vi "Logic.vi"(8 "error in (no error)":errorcluster, 11 "CIFPlugin in":refnum<class "Template_Plugin.lvclass">) -> (0 "error out":errorcluster, 3 "CIFPlugin out":refnum<class "Template_Plugin.lvclass">)   [LabVIEW 2021, in "Template_Plugin.lvclass"]
uses:
  Template_Plugin.lvclass
  <vilib>/CIF Foundation/CIF Core/CIFCore/Class/CIFCorePlugin.lvclass
  Common/Typedef/Channels.ctl
  Common/Template_Common.lvlib
  C:/Program Files/National Instruments/LabVIEW 2021/vi.lib/CIF Foundation/CIF Core/CIFCore/Class/CIFCorePlugin.lvclass
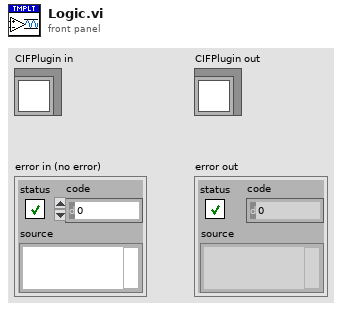
[diagram p1: front panel]
types:
  T1 = typedef "Template_Common.lvlib/Channels.ctl" = enum16{"doubleout", "doublein1", "doublein2", "uint_out", "uint_in"}
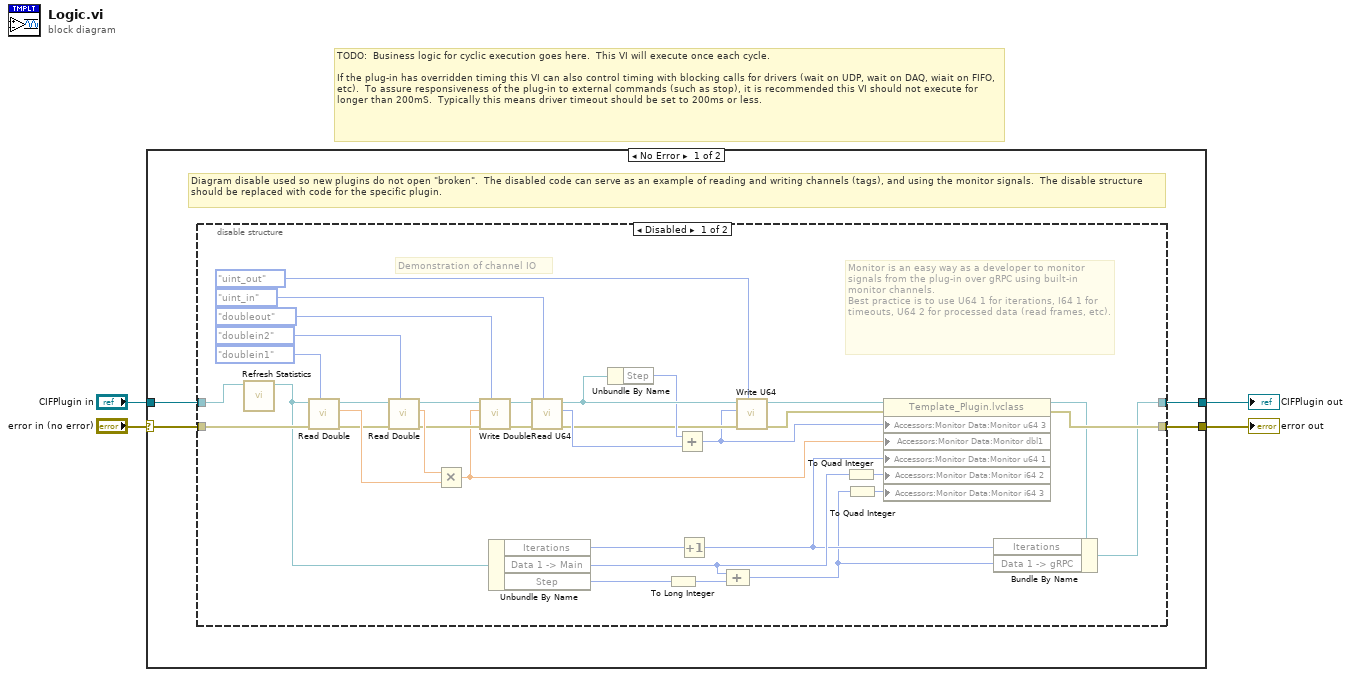
[diagram p0: block diagram]
diagram:
  # "TODO:  Business logic for cyclic execution goes here.  This VI will execute once each cycle.  \n\nIf the plug-in has overridden timing this VI can also control timing with blocking calls for drivers (wait on UDP, wait on DAQ, wiait on FIFO, etc).  To assure responsiveness of the plug-in to external commands (such as stop), it is recommended this VI should not execute for longer than 200mS.  Typically this means driver timeout should be set to 200ms or less."
  n1 = case shown="No Error" "error in (no error)" {
    selector: "error in (no error)" -> [w5 w47]
    tunnel: [w8 w47] -> w2
    tunnel: [w7 w46] -> w1
    tunnel: "CIFPlugin in" -> [w6 w46]
    frame No Error {
      # "Diagram disable used so new plugins do not open \"broken\".  The disabled code can serve as an example of reading and writing channels (tags), and using the monitor signals.  The disable structure should be replaced with code for the specific plugin."
      n2 = disable-structure shown="Disabled" {
        disable-tunnel: [w43 w44] -> w8
        disable-tunnel: [w36 w45] -> w7
        disable-tunnel: w6 -> [w10 w45]
        disable-tunnel: w5 -> [w16 w44]
        frame Disabled {
          # "Demonstration of channel IO"
          # "Monitor is an easy way as a developer to monitor signals from the plug-in over gRPC using built-in monitor channels.  \nBest practice is to use U64 1 for iterations, I64 1 for timeouts, U64 2 for processed data (read frames, etc)."
          n3 = call "Refresh Statistics.vi"("CIFPlugin in"=w10) -> ("CIFPlugin out"=w9:refnum<class "Template_Plugin.lvclass">)  [unwired: 10 in]
          n4 = call <vilib>:"Read Double.vi"("Channel Index"=Channels."doublein1" ("Channels"), "error in (no error)"=w16, "CIFCorePlugin in"=w9) -> ("error out"=w26:errorcluster, "Data"=w27:dbl, "CIFCorePlugin out"=w25:refnum<class "Template_Plugin.lvclass">)  [unwired: 6 in]
          n5 = call <vilib>:"Read Double.vi"("Channel Index"=Channels."doublein2" ("Channels"), "error in (no error)"=w26, "CIFCorePlugin in"=w25) -> ("error out"=w23:errorcluster, "Data"=w24:dbl, "CIFCorePlugin out"=w22:refnum<class "Template_Plugin.lvclass">)  [unwired: 6 in]
          n6 = Multiply(x=w24, y=w27) -> (x*y=w14:dbl)
          n7 = call <vilib>:"Write Double.vi"("Channel Index"=Channels."doubleout" ("Channels"), "error in (no error)"=w23, "Data"=w14, "CIFCorePlugin in"=w22) -> ("error out"=w20:errorcluster, "CIFCorePlugin out"=w21:refnum<class "Template_Plugin.lvclass">)  [unwired: 6 in]
          n8 = Unbundle By Name(w9) -> ("Iterations"=w15:u64, "Data 1 -> Main"=w40:i32, "Step"=w34:u64)
          n9 = call <vilib>:"Read U64.vi"("Channel Index"=Channels."uint_in" ("Channels"), "error in (no error)"=w20, "CIFCorePlugin in"=w21) -> ("error out"=w18:errorcluster, "Data"=w32:u64, "CIFCorePlugin out"=w33:refnum<class "Template_Plugin.lvclass">)  [unwired: 6 in]
          n10 = Unbundle By Name(w33) -> ("Step"=w31:u64)
          n11 = To Long Integer(number=w34) -> (32bit integer=w41:i32)
          n12 = Add(x=w31, y=w32) -> (x+y=w13:u64)
          n13 = Increment(x=w15) -> (x+1=w12:u64)
          n14 = Compound Arithmetic op=ADD(w40, w41) -> (w11:i32)
          n15 = call <vilib>:"Write U64.vi"("Channel Index"=Channels."uint_out" ("Channels"), "error in (no error)"=w18, "Data"=w13, "CIFCorePlugin in"=w33) -> ("error out"=w19:errorcluster, "CIFCorePlugin out"=w17:refnum<class "Template_Plugin.lvclass">)  [unwired: 6 in]
          n16 = To Quad Integer(1:w40) -> (0:w39:i64)
          n17 = To Quad Integer(1:w11) -> (0:w38:i64)
          n18 = property class="Template_Plugin.lvclass"(reference=w17, error in=w19, "Accessors:Monitor Data:Monitor u64 3"=w13, "Accessors:Monitor Data:Monitor dbl1"=w14, "Accessors:Monitor Data:Monitor u64 1"=w12, "Accessors:Monitor Data:Monitor i64 2"=w39, "Accessors:Monitor Data:Monitor i64 3"=w38) -> (reference out=w37:refnum<class "Template_Plugin.lvclass">, error out=w43:errorcluster)
          n19 = Bundle By Name(cluster=w37, "Iterations"=w12, "Data 1 -> gRPC"=w11) -> (w36:refnum<class "Template_Plugin.lvclass">)
        }
        frame Enabled {
        }
      }
    }
    frame Error {
    }
  }
  "error out" <- w2
  "CIFPlugin out" <- w1
